vi "read_attributes.vi"(8 "error in (no error)":errorcluster caption="entrée d'erreur (pas d'erreur)", 11 "LogisticRegression en entrée":refnum<class "LogisticRegression.lvclass">) -> (0 "error out":errorcluster caption="sortie d'erreur", 2 "attributes":T1, 3 "LogisticRegression en sortie":refnum<class "LogisticRegression.lvclass">)   [LabVIEW 2020, in "LogisticRegression.lvclass"]
uses:
  LogisticRegression.lvclass
  Controls/logistic_regression_attributes.ctl
  LogisticRegression.lvclass/LogisticRegression.ctl
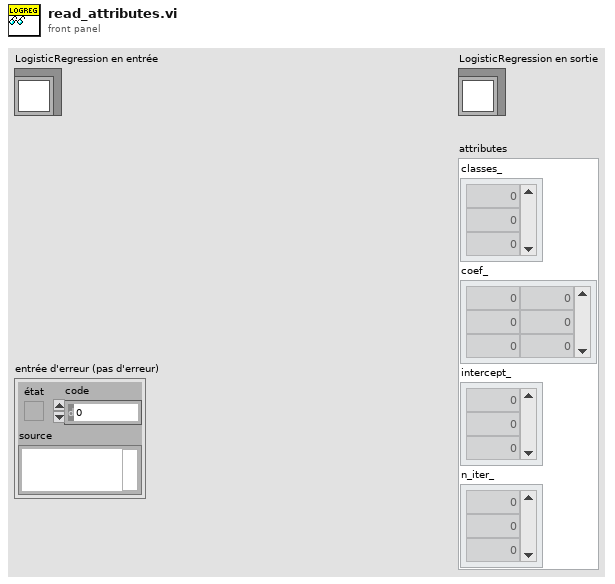
[diagram p1: front panel]
types:
  T1 = typedef "logistic_regression_attributes.ctl" = cluster{"classes_":dbl[], "coef_":dbl[][], "intercept_":dbl[], "n_iter_":dbl[]}
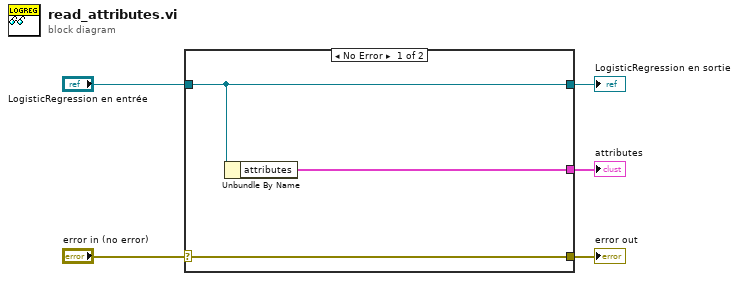
[diagram p0: block diagram]
diagram:
  n1 = case shown="No Error" "error in (no error)" {
    selector: "error in (no error)" -> [w8 w9]
    tunnel: [w8 w9] -> w4
    tunnel: [w7 w10] -> w2
    tunnel: "LogisticRegression en entrée" -> [w7 w10]
    tunnel: [w6 _] -> w1
    frame No Error {
      n2 = Unbundle By Name(w7) -> ("attributes"=w6:T1)
    }
    frame Error {
    }
  }
  "error out" <- w4
  "LogisticRegression en sortie" <- w2
  "attributes" <- w1
